vi "DFTV2.vi"(8 "error in (no error)":errorcluster, 11 "ChirpV2 in":refnum<class "ChirpV2.lvclass">) -> (0 "error out":errorcluster, 3 "ChirpV2 out":refnum<class "ChirpV2.lvclass">)   [LabVIEW 2014, in "ChirpV2.lvclass"]
uses:
  ChirpV2.lvclass
  <vilib>/Analysis/2dsp.llb/Real FFT.vi
  <vilib>/Analysis/NI_AALPro.lvlib
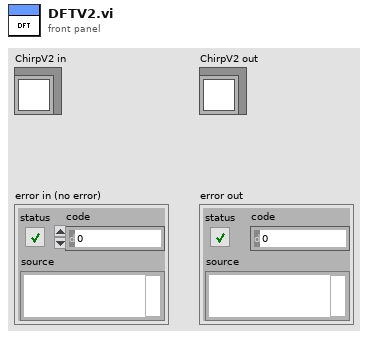
[diagram p1: front panel]
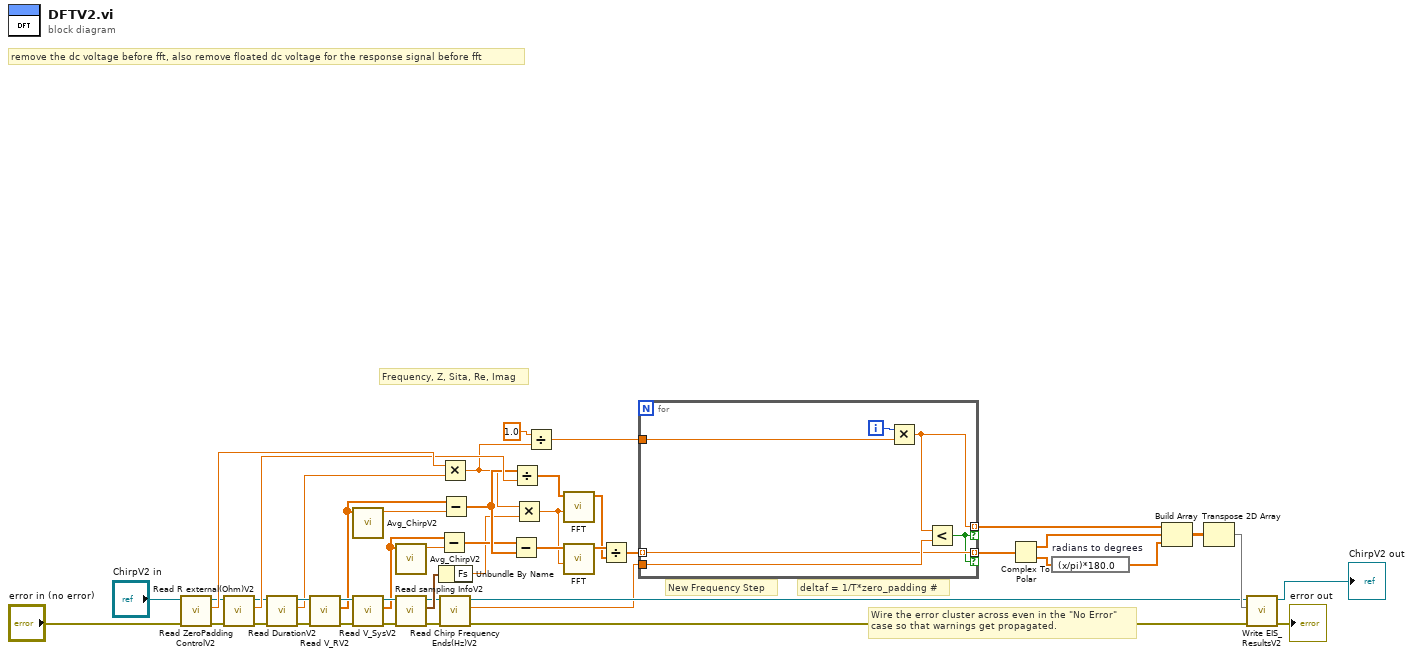
[diagram p0: block diagram]
diagram:
  # "deltaf = 1/T*zero_padding #"
  # "remove the dc voltage before fft, also remove floated dc voltage for the response signal before fft"
  # "Frequency, Z, Sita, Re, Imag"
  # "New Frequency Step"
  # "Wire the error cluster across even in the \"No Error\"\ncase so that warnings get propagated."
  n1 = call-dynamic "Read ZeroPadding ControlV2.vi"("error in (no error)"="error in (no error)", "ChirpV2 in"="ChirpV2 in") -> ("error out"=w45:errorcluster, "ZeroPadding Control"=w46:dbl, "ChirpV2 out"=w44:refnum<class "ChirpV2.lvclass">)  [unwired: 7 in]
  n2 = call-dynamic "Read R external(Ohm)V2.vi"("error in (no error)"=w45, "ChirpV2 in"=w44) -> ("error out"=w21:errorcluster, "R external(Ohm)"=w36:dbl, "ChirpV2 out"=w23:refnum<class "ChirpV2.lvclass">)  [unwired: 7 in]
  n3 = call-dynamic "Read DurationV2.vi"("error in (no error)"=w21, "ChirpV2 in"=w23) -> ("error out"=w20:errorcluster, "Duration"=w19:dbl, "ChirpV2 out"=w22:refnum<class "ChirpV2.lvclass">)  [unwired: 7 in]
  n4 = call-dynamic "Read V_RV2.vi"("error in (no error)"=w20, "ChirpV2 in"=w22) -> ("error out"=w38:errorcluster, "V_R"=w4:dbl[], "ChirpV2 out"=w37:refnum<class "ChirpV2.lvclass">)  [unwired: 7 in]
  n5 = call "Avg_ChirpV2.vi"("Array"=w4) -> ("Avg"=w3:dbl)  [unwired: 10 in]
  n6 = call-dynamic "Read V_SysV2.vi"("error in (no error)"=w38, "ChirpV2 in"=w37) -> ("error out"=w17:errorcluster, "V_Sys"=w2:dbl[], "ChirpV2 out"=w18:refnum<class "ChirpV2.lvclass">)  [unwired: 7 in]
  n7 = call "Avg_ChirpV2.vi"("Array"=w2) -> ("Avg"=w1:dbl)  [unwired: 10 in]
  n8 = call-dynamic "Read sampling InfoV2.vi"("error in (no error)"=w17, "ChirpV2 in"=w18) -> ("error out"=w11:errorcluster, "sampling Info"=w16:cluster{"Fs":dbl}, "ChirpV2 out"=w12:refnum<class "ChirpV2.lvclass">)  [unwired: 7 in]
  n9 = Subtract(x=w2, y=w1) -> (x-y=w34:dbl[])
  n10 = Unbundle By Name(w16) -> ("Fs"=w14:dbl)
  n11 = Multiply(x=w46, y=w19) -> (x*y=w15:dbl)
  n12 = call-dynamic "Read Chirp Frequency Ends(Hz)V2.vi"("error in (no error)"=w11, "ChirpV2 in"=w12) -> ("error out"=w9:errorcluster, "Chirp Frequency Ends(Hz)"=w8:dbl, "ChirpV2 out"=w10:refnum<class "ChirpV2.lvclass">)  [unwired: 7 in]
  n13 = Subtract(x=w4, y=w3) -> (x-y=w35:dbl[])
  n14 = Subtract(x=w34, y=w35) -> (x-y=w24:dbl[])
  n15 = Divide(x=w35, y=w36) -> (x/y=w27:dbl[])
  n16 = Multiply(x=w15, y=w14) -> (x*y=w13:dbl)
  n17 = Divide(x=1.0, y=w15) -> (x/y=w7:dbl)
  n18 = call-poly <vilib>:"FFT.vi"("FFT size"=w13, "X"=w27) -> ("FFT {X}"=w25:cdb[])  [unwired: 8 in, 1 out]
  n19 = call-poly <vilib>:"FFT.vi"("FFT size"=w13, "X"=w24) -> ("FFT {X}"=w26:cdb[])  [unwired: 8 in, 1 out]
  n20 = Divide(x=w26, y=w25) -> (x/y=w6:cdb[])
  n21 = for {
    tunnel: w7 -> [w52]
    tunnel: [w50] -> w30 mode=indexing if=w47
    tunnel: w8 -> [w49]
    tunnel: w6 -> [w48] mode=indexing
    tunnel: [w48] -> w5 mode=indexing if=w47
    i -> [w51]
    n22 = Multiply(x=w51, y=w52) -> (x*y=w50:dbl)
    n23 = Less?(x=w50, y=w49) -> (x < y?=w47:bool)
  }
  n24 = Complex To Polar(r * e^(i*theta)=w5) -> (r=w29:dbl[], theta=w32:dbl[])
  n25 = expression code="(x/pi)*180.0" "radians to degrees"(w32) -> (w33:dbl[])
  n26 = Build Array(w30, w29, w33) -> (w28:dbl[][])
  n27 = Transpose 2D Array(2D array=w28) -> (transposed array=w39:dbl[][])
  n28 = call-dynamic "Write EIS_ResultsV2.vi"("error in (no error)"=w9, "EIS_Results"=w39, "ChirpV2 in"=w10) -> ("error out"=→"error out":errorcluster, "ChirpV2 out"=→"ChirpV2 out":refnum<class "ChirpV2.lvclass">)  [unwired: 7 in]
